vi "CAL-Save Data.vi"(0 "path":path, 5 "Data":T1, 7 "Stimulus":T4={"Type"="", "Freq step (Hz)"=50.0, "Sampling rate (Hz)"=50000.0, "Attenuation (dB)"=20.0}, 9 "Response":T2, 11 "error in (no error)":errorcluster, 12 "Backup folder":string) -> (4 "new file path":path, 15 "error out":errorcluster)   [LabVIEW 2020]
uses:
  Typedefs/CAL-Stimulus.ctl
  Typedefs/CAL-Response.ctl
  Typedefs/CAL-Data.ctl
  Typedefs/CAL-Globals.vi
panel:
  in  "ACOUSTIC CALIBRATION":T3
  in  "backup":bool=TRUE
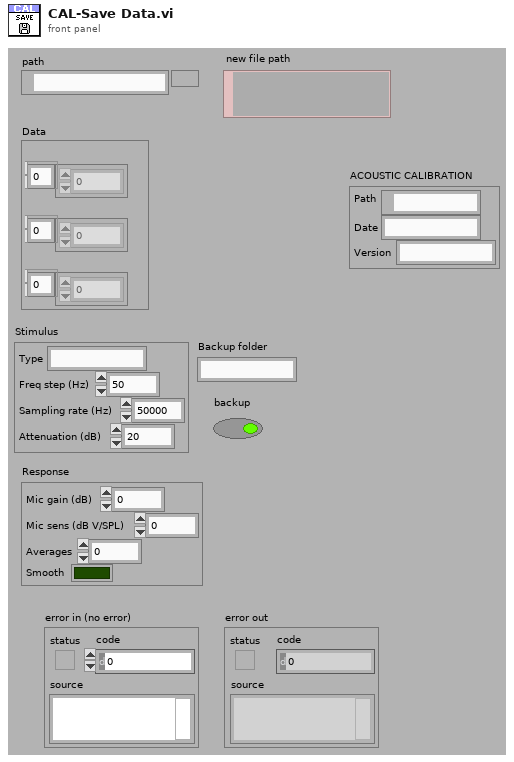
[diagram p1: front panel]
types:
  T1 = typedef "CAL-Data.ctl" = cluster{"Freq (Hz)":dbl[], "Magnitude (dB SPL/V)":dbl[], "Phase (degrees)":dbl[]}
  T2 = typedef "CAL-Response.ctl" = cluster{"Mic gain (dB)":dbl, "Mic sens (dB V/SPL)":dbl, "Averages":i32, "Smooth":bool}
  T3 = cluster{"Path":path, "Date":string, "Version":string}
  T4 = typedef "CAL-Stimulus.ctl" = cluster{"Type":string, "Freq step (Hz)":dbl, "Sampling rate (Hz)":dbl, "Attenuation (dB)":dbl}
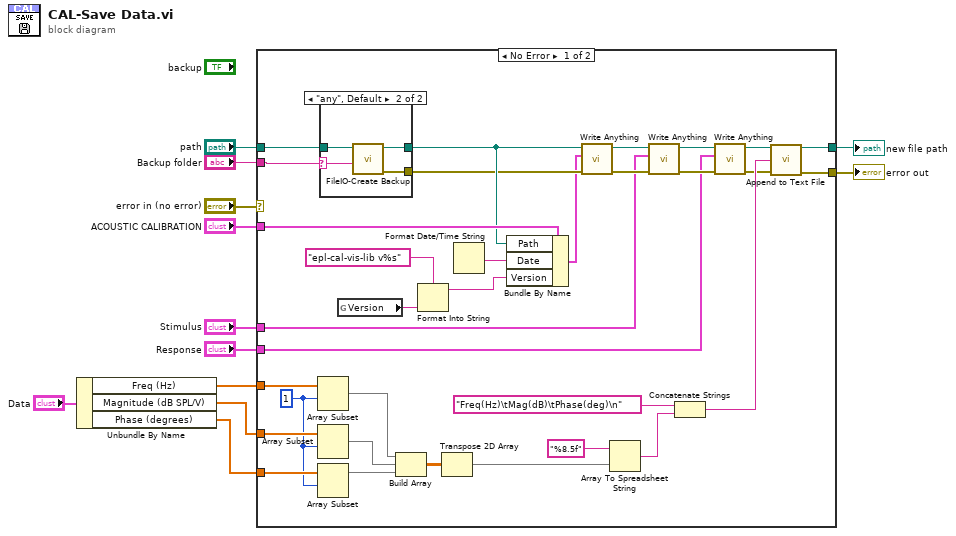
[diagram p0: block diagram]
diagram:
  n1 = Unbundle By Name("Data") -> ("Freq (Hz)"=w3:dbl[], "Magnitude (dB SPL/V)"=w2:dbl[], "Phase (degrees)"=w1:dbl[])
  n2 = case shown="No Error" "error in (no error)" {
    selector: "error in (no error)" -> [_ w51]
    tunnel: w1 -> [w45 _]
    tunnel: w2 -> [w44 _]
    tunnel: w3 -> [w40 _]
    tunnel: [w22 w51] -> w12
    tunnel: "Stimulus" -> [w26 _]
    tunnel: "path" -> [w35 _]
    tunnel: "Backup folder" -> [w34 _]
    tunnel: "ACOUSTIC CALIBRATION" -> [w33 _]
    tunnel: [w21 _] -> w6
    tunnel: "Response" -> [w16 _]
    frame No Error {
      w37 = 1 ("index")
      n3 = Array Subset(array=w40, index=w37) -> (w36:dbl[])  [unwired: 1 in]
      n4 = Array Subset(array=w44, index=w37) -> (w39:dbl[])  [unwired: 1 in]
      n5 = Array Subset(array=w45, index=w37) -> (w38:dbl[])  [unwired: 1 in]
      n6 = case shown="\"any\", Default" w34 {
        selector: w34 -> [_ w47]
        tunnel: w35 -> [w46 w50]
        tunnel: [w46 w49] -> w31
        tunnel: [_ w48] -> w30
        frame "" {
        }
        frame "any", Default {
          n7 = call "FileIO-Create Backup.vi"("Subfolder"=w47, "Path"=w50) -> ("error out"=w48:errorcluster, "Path (thru)"=w49:path)  [unwired: 6 in, 2 out]
        }
      }
      n8 = global read "CAL-Globals.vi" "Version"() -> (w15:string)
      n9 = Build Array(w36, w39, w38) -> (w42:dbl[][])
      n10 = Format Into String(format string="epl-cal-vis-lib v%s", w15) -> (resulting string=w13:string)  [unwired: 2 in, 1 out]
      n11 = Transpose 2D Array(2D array=w42) -> (transposed array=w41:dbl[][])
      n12 = Format Date/Time String() -> (date/time string=w32:string)  [unwired: 3 in]
      n13 = Bundle By Name(cluster=w33, "Path"=w31, "Date"=w32, "Version"=w13) -> (w29:T3)
      n14 = call "Write Anything.vi"("Error In"=w30, "Anything"=w29, "Path (dialog)"=w31) -> ("Error Out"=w27:errorcluster, "Path out"=w28:path)  [unwired: 7 in]
      n15 = Array To Spreadsheet String(array=w41, 3:"%8.5f" ("format (%.3f)")) -> (spreadsheet string=w24:string)  [unwired: 1 in]
      n16 = call "Write Anything.vi"("Error In"=w27, "Anything"=w26, "Path (dialog)"=w28) -> ("Error Out"=w17:errorcluster, "Path out"=w20:path)  [unwired: 7 in]
      n17 = Concatenate Strings("Freq(Hz)\tMag(dB)\tPhase(deg)\n" ("format string"), w24) -> (w23:string)
      n18 = call "Write Anything.vi"("Error In"=w17, "Anything"=w16, "Path (dialog)"=w20) -> ("Error Out"=w18:errorcluster, "Path out"=w19:path)  [unwired: 7 in]
      n19 = call "Append to Text File.vi"("file path"=w19, "text"=w23, "error in (no error)"=w18) -> ("file path out"=w21:path, "error out"=w22:errorcluster)  [unwired: 11 in]
    }
    frame Error {
    }
  }
  "error out" <- w12
  "new file path" <- w6
